vi "ToTable.vi"(8 "error in":errorcluster, 9 "Table Index (0)":i32, 10 "variant":variant, 11 "SQLite editor node in":refnum<class "SQLite editor node.lvclass">) -> (0 "error out":errorcluster, 1 "row headers":string[](array[string]), 2 "table":string[][](array[string]), 3 "SQLite editor node out":refnum<class "SQLite editor node.lvclass">)   [LabVIEW 2014, in "SQLite editor node.lvclass"]
doc: "Generates the strings needed to display on a table based on the information found in the engine and module configuration classes."
uses:
  SQLite editor node.lvclass
  module/configuration/SQLite configuration.lvclass
  <vilib>/NI/Module Execution Interface/Engine Configuration/engine configuration.lvclass
  module/configuration/SQLite configuration.lvclass/SQLite configuration.ctl
  <vilib>/NI/Configuration Framework/serializable configuration/NISE_CEF_serializable configuration.lvclass/NISE_CEF_serializable configuration.ctl
  <vilib>/NI/Tag Bus/tag/tag descriptor.lvclass/tag descriptor.ctl
  <vilib>/NI/Tag Bus Module Framework/channel/TBM channel.lvclass/TBM channel.ctl
  module/configuration/Read Lines.vi
  <vilib>/Utility/LVClass/Get LV Class Name.vi
  <vilib>/NI/Configuration Framework/error generator/NISE_error generator.vi
  <vilib>/NI/Tag Bus Module Framework/channel/TBM channel.lvclass
  <vilib>/NI/Tag Bus/tag/tag descriptor.lvclass
  <vilib>/NI/Configuration Framework/serializable configuration/NISE_CEF_serializable configuration.lvclass
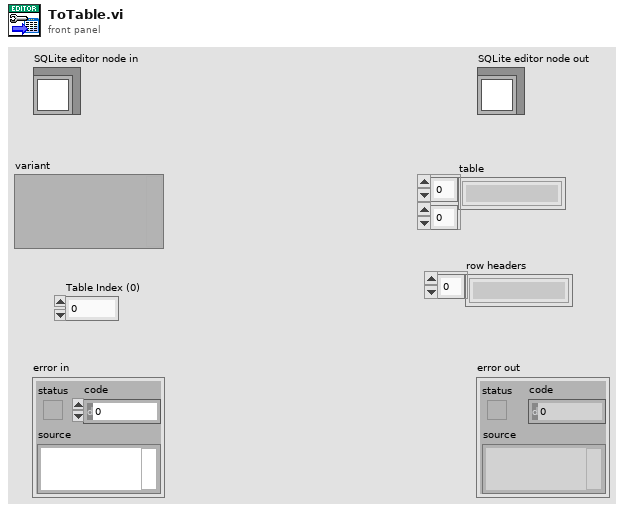
[diagram p1: front panel]
types:
  T1 = typedef "tag bus configurable plugin module configuration.lvclass/Line.ctl" = cluster{"channel":refnum<class "TBM channel.lvclass">}
  T2 = typedef "TBM channel.lvclass/channel classification.ctl" = enum16{"input data", "output data", "processing parameter", "processing result"}
  T3 = typedef "tag bus.lvlib/tag descriptor.lvclass/Data Type.ctl" = enum16{"Double", "Single", "I64", "I32", "I16", "I8", "U64", "U32", "U16", "U8", "Boolean", "String", "Array of Double", "Array of Single", "Array of I64", "Array of I32", "Array of I16", "Array of I8", "Array of U64", "Array of U32", "Array of U16", "Array of U8", "Array of Boolean", "Array of String"}
  T4 = typedef "SQLite editor node.lvclass/permissions.ctl" = enum32{"Read from DB", "Write to DB"}
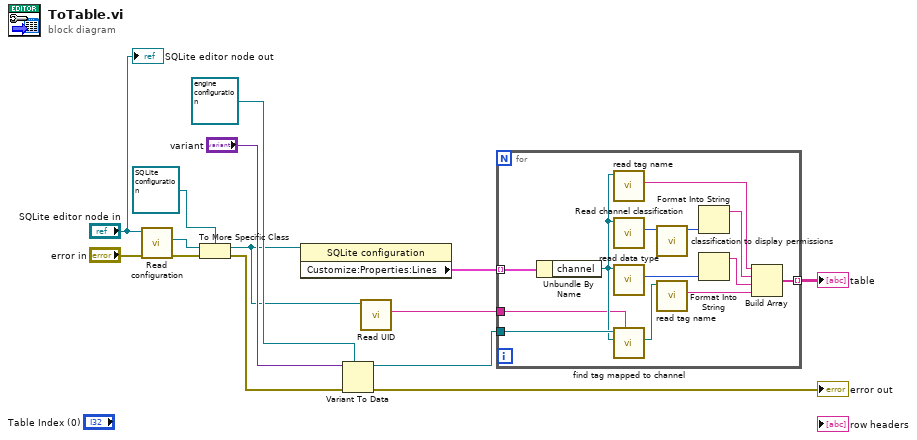
[diagram p0: block diagram]
diagram:
  n1 = call-dynamic "Read configuration.vi"("error in"="error in", "SQLite editor node in"="SQLite editor node in") -> ("error out"=w14:errorcluster, "configuration"=w5:refnum<class "NISE_CEF_serializable configuration.lvclass">)  [unwired: 7 in, 1 out]
  n2 = To More Specific Class(target class=refnum<class "SQLite configuration.lvclass"> refnum ("tag bus configurable plugin module configuration"), reference=w5, error in=w14) -> (specific class reference=w4:refnum<class "SQLite configuration.lvclass">, error out=w2:errorcluster)
  n3 = property class="SQLite configuration"(reference=w4) -> ("Customize:Properties:Lines"=w11:T1[])  [unwired: 1 in, 2 out]
  n4 = Variant To Data(error in=w2, type=refnum<class "engine configuration.lvclass"> refnum ("engine configuration"), Variant="variant") -> (data=w8:refnum<class "engine configuration.lvclass">, error out=→"error out":errorcluster)
  n5 = call <vilib>:"Read UID.vi"("configuration in"=w4) -> ("instance id"=w3:string)  [unwired: 8 in, 2 out]
  n6 = for {
    tunnel: w11 -> [w27] mode=indexing
    tunnel: w8 -> [w25]
    tunnel: [w16] -> w6 mode=indexing
    tunnel: w3 -> [w15]
    n7 = Unbundle By Name(w27) -> ("channel"=w19:refnum<class "TBM channel.lvclass">)
    n8 = call <vilib>:"read tag name.vi"("system tag in"=w19) -> ("name"=w26:string)  [unwired: 8 in, 2 out]
    n9 = call <vilib>:"Read channel classification.vi"("channel in"=w19) -> ("channel classification"=w23:T2)  [unwired: 8 in, 2 out]
    n10 = call <vilib>:"read data type.vi"("system tag in"=w19) -> ("data type"=w18:T3)  [unwired: 8 in, 2 out]
    n11 = call <vilib>:"find tag mapped to channel.vi"("owner"=w15, "channel"=w19, "engine configuration in"=w25) -> ("tag"=w24:refnum<class "tag descriptor.lvclass">)  [unwired: 6 in, 2 out]
    n12 = call "classification to display permissions.vi"("channel classification"=w23) -> ("permissions"=w22:T4)  [unwired: 10 in]
    n13 = call <vilib>:"read tag name.vi"("system tag in"=w24) -> ("name"=w20:string)  [unwired: 8 in, 2 out]
    n14 = Format Into String(w22) -> (resulting string=w21:string)  [unwired: 3 in, 1 out]
    n15 = Format Into String(w18) -> (resulting string=w17:string)  [unwired: 3 in, 1 out]
    n16 = Build Array(w26, w21, w17, w20) -> (w16:string[])
  }
  "table" <- w6
  "SQLite editor node out" <- "SQLite editor node in"
